vi "Test MQTT-3.1.3-10.vi"(8 "error in (no error)":errorcluster) -> (0 "error out":errorcluster)   [LabVIEW 2013]
uses:
  source/Control Packets/CONNECT/ConnectFlags -- cluster.ctl
  <vilib>/addons/_JKI Toolkits/Caraya/classes/Assert/Assert Equal Value_Variant.vi
  <vilib>/addons/_JKI Toolkits/Caraya/classes/Assert/Assert Greater_Variant.vi
  source/Control Packets/CONNECT/CONNECT.lvclass
  <vilib>/addons/_JKI Toolkits/Caraya/classes/Test/Test.lvclass
  source/Control Packets/ControlPacket/ControlPacket.lvclass
  <vilib>/addons/_JKI Toolkits/Caraya/classes/Assert/Assert.lvclass
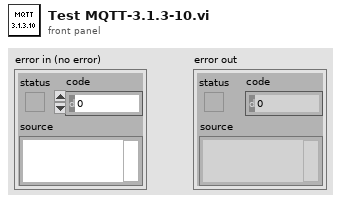
[diagram p1: front panel]
types:
  T1 = cluster{"Will Topic":string, "Will Message":string, "Username":string, "Password":string}
  T2 = typedef "CONNECT.lvclass/ConnectFlags -- cluster.ctl" = cluster{"Reserved":bool, "Clean Session":bool, "Will Flag":bool, "Will QoS 1":bool, "Will QoS 2":bool, "Will Retain":bool, "Password Flag":bool, "User Name Flag":bool}
  T3 = typedef "CONNECT.lvclass/ConnectPayload -- cluster.ctl" = cluster{"Will Topic":string, "Will Message":string, "Username":string, "Password":string}
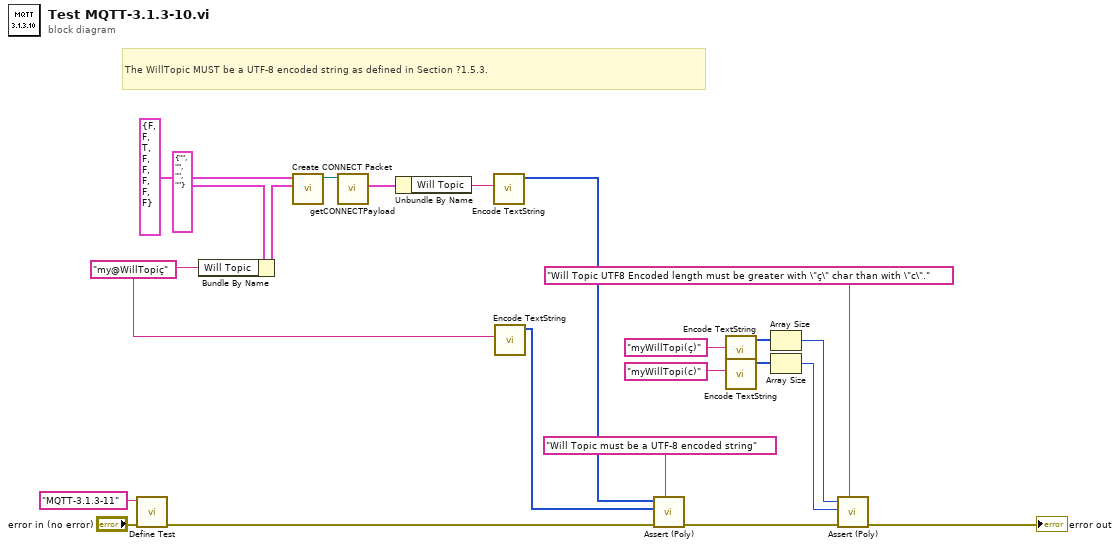
[diagram p0: block diagram]
diagram:
  w12 = "my@WillTopiç" ("Username")
  # "The WillTopic MUST be a UTF-8 encoded string as defined in Section ?1.5.3."
  n1 = call <vilib>:"Define Test.vi"("error in (no error)"="error in (no error)", "Label (VI Title)"="MQTT-3.1.3-11") -> ("error out"=w19:errorcluster)  [unwired: 9 in]
  n2 = Bundle By Name(cluster=T1 {"Will Topic"="", "Will Message"="", "Username"="", "Password"=""} ("Payload"), "Will Topic"=w12) -> (w14:T1)
  n3 = call "Create CONNECT Packet.vi"("Payload"=w14, "Connect Flags"=T2 {"Reserved"=FALSE, "Clean Session"=FALSE, "Will Flag"=TRUE, "Will QoS 1"=FALSE, "Will QoS 2"=FALSE, "Will Retain"=FALSE, "Password Flag"=FALSE, "User Name Flag"=FALSE}) -> ("CONNECT"=w17:refnum<class "CONNECT.lvclass">)  [unwired: 8 in, 1 out]
  n4 = call "getCONNECTPayload.vi"("CONNECT in"=w17) -> ("Payload"=w16:T3)  [unwired: 9 in, 1 out]
  n5 = Unbundle By Name(w16) -> ("Will Topic"=w13:string)
  n6 = call "Encode TextString.vi"("Text String"=w13) -> ("Length-Prefixed Field"=w10:u8[])  [unwired: 10 in]
  n7 = call "Encode TextString.vi"("Text String"=w12) -> ("Length-Prefixed Field"=w11:u8[])  [unwired: 10 in]
  n8 = call-poly <vilib>:"Assert (Poly).vi"("Label"="Will Topic must be a UTF-8 encoded string", "error in (no error)"=w19, "Y"=w11, "X"=w10) -> ("error out"=w9:errorcluster)  [unwired: 7 in]
  n9 = call "Encode TextString.vi"("Text String"="myWillTopi(ç)" ("Username")) -> ("Length-Prefixed Field"=w4:u8[])  [unwired: 10 in]
  n10 = call "Encode TextString.vi"("Text String"="myWillTopi(c)" ("Username")) -> ("Length-Prefixed Field"=w3:u8[])  [unwired: 10 in]
  n11 = Array Size(array=w4) -> (size(s)=w1:i32)
  n12 = Array Size(array=w3) -> (size(s)=w2:i32)
  n13 = call-poly <vilib>:"Assert (Poly).vi"("Label"="Will Topic UTF8 Encoded length must be greater with \"ç\" char than with \"c\".", "error in (no error)"=w9, "Y"=w2, "X"=w1) -> ("error out"=→"error out":errorcluster)  [unwired: 7 in]
